vi "Translate Weight Calibration.vi"(10 "Known Weight Tool Coordinates":T1, 11 "Known HDI Fiducials Coordinates":T2) -> (1 "brass piece rotation":dbl, 2 "Orient3d String":string, 3 "Vec3d String":string)   [LabVIEW 2011]
uses:
  Shared Components/Vec3d Class/Vec3d Class.lvclass
  Shared Components/Orient3d Class/Orient3d Class.lvclass
panel:
  out "Pos Z":dbl
  out "Pos Y":dbl
  out "Pos X":dbl
  out "orient w":dbl
  out "orient z":dbl
  out "orient y":dbl
  out "orient x":dbl
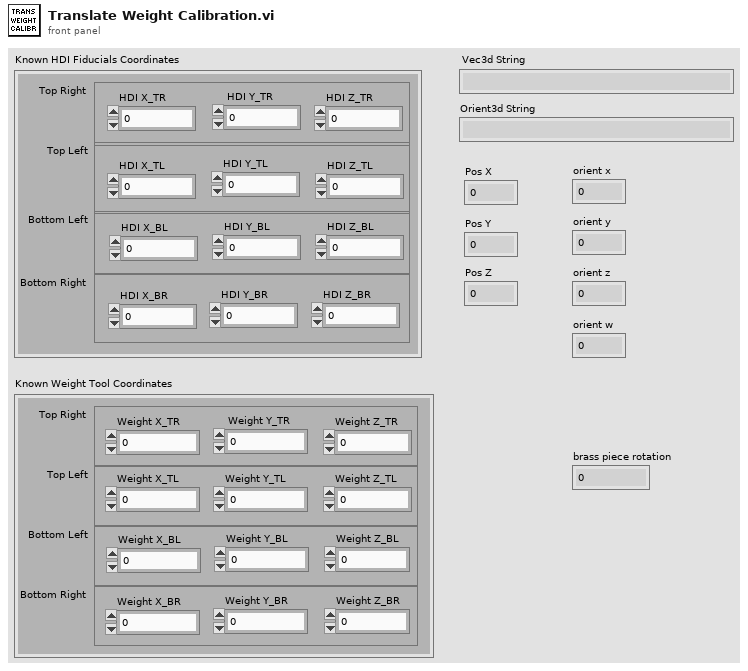
[diagram p1: front panel]
types:
  T1 = cluster{"Top Right":cluster{"Weight X_TR":dbl, " Weight Y_TR":dbl, "Weight Z_TR":dbl}, "Top Left":cluster{"Weight X_TL":dbl, "Weight Y_TL":dbl, "Weight Z_TL":dbl}, "Bottom Left":cluster{"Weight X_BL":dbl, "Weight Y_BL":dbl, "Weight Z_BL":dbl}, "Bottom Right":cluster{"Weight X_BR":dbl, "Weight Y_BR":dbl, "Weight Z_BR":dbl}}
  T2 = cluster{"Top Right":cluster{"HDI X_TR":dbl, " HDI Y_TR":dbl, "HDI Z_TR":dbl}, "Top Left":cluster{"HDI X_TL":dbl, "HDI Y_TL":dbl, "HDI Z_TL":dbl}, "Bottom Left":cluster{"HDI X_BL":dbl, "HDI Y_BL":dbl, "HDI Z_BL":dbl}, "Bottom Right":cluster{"HDI X_BR":dbl, "HDI Y_BR":dbl, "HDI Z_BR":dbl}}
  T3 = cluster{"Weight X_TR":dbl, " Weight Y_TR":dbl, "Weight Z_TR":dbl}
  T4 = cluster{"Weight X_TL":dbl, "Weight Y_TL":dbl, "Weight Z_TL":dbl}
  T5 = cluster{"Weight X_BL":dbl, "Weight Y_BL":dbl, "Weight Z_BL":dbl}
  T6 = cluster{"Weight X_BR":dbl, "Weight Y_BR":dbl, "Weight Z_BR":dbl}
  T7 = cluster{"HDI X_TR":dbl, " HDI Y_TR":dbl, "HDI Z_TR":dbl}
  T8 = cluster{"HDI X_TL":dbl, "HDI Y_TL":dbl, "HDI Z_TL":dbl}
  T9 = cluster{"HDI X_BL":dbl, "HDI Y_BL":dbl, "HDI Z_BL":dbl}
  T10 = cluster{"HDI X_BR":dbl, "HDI Y_BR":dbl, "HDI Z_BR":dbl}
  T11 = typedef "Position_Orientation.ctl" = cluster{"Center":refnum<class "Vec3d Class.lvclass">, "Orientation":refnum<class "Orient3d Class.lvclass">}
  T12 = typedef "Quaternion.ctl" = cluster{"x":dbl, "y":dbl, "z":dbl, "w":dbl}
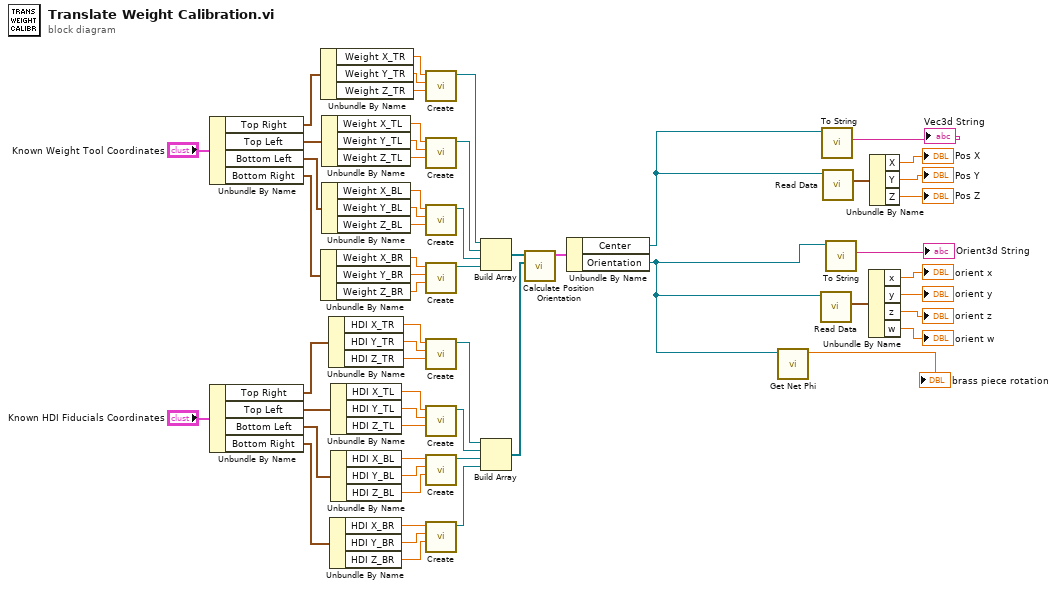
[diagram p0: block diagram]
diagram:
  n1 = Unbundle By Name("Known Weight Tool Coordinates") -> ("Top Right"=w22:T3, "Top Left"=w21:T4, "Bottom Left"=w20:T5, "Bottom Right"=w19:T6)
  n2 = Unbundle By Name("Known HDI Fiducials Coordinates") -> ("Top Right"=w39:T7, "Top Left"=w35:T8, "Bottom Left"=w28:T9, "Bottom Right"=w24:T10)
  n3 = Unbundle By Name(w22) -> ("Weight X_TR"=w18:dbl, "Weight Y_TR"=w17:dbl, "Weight Z_TR"=w16:dbl)
  n4 = Unbundle By Name(w19) -> ("Weight X_BR"=w9:dbl, "Weight Y_BR"=w8:dbl, "Weight Z_BR"=w7:dbl)
  n5 = Unbundle By Name(w21) -> ("Weight X_TL"=w15:dbl, "Weight Y_TL"=w14:dbl, "Weight Z_TL"=w13:dbl)
  n6 = Unbundle By Name(w20) -> ("Weight X_BL"=w12:dbl, "Weight Y_BL"=w11:dbl, "Weight Z_BL"=w10:dbl)
  n7 = Unbundle By Name(w39) -> ("HDI X_TR"=w38:dbl, "HDI Y_TR"=w37:dbl, "HDI Z_TR"=w36:dbl)
  n8 = Unbundle By Name(w24) -> ("HDI X_BR"=w27:dbl, "HDI Y_BR"=w26:dbl, "HDI Z_BR"=w25:dbl)
  n9 = Unbundle By Name(w35) -> ("HDI X_TL"=w34:dbl, "HDI Y_TL"=w33:dbl, "HDI Z_TL"=w32:dbl)
  n10 = Unbundle By Name(w28) -> ("HDI X_BL"=w31:dbl, "HDI Y_BL"=w30:dbl, "HDI Z_BL"=w29:dbl)
  n11 = call "Create.vi"("Z"=w16, "Y"=w17, "X"=w18) -> ("Vec3d Class out"=w55:refnum<class "Vec3d Class.lvclass">)  [unwired: 7 in, 1 out]
  n12 = call "Create.vi"("Z"=w13, "Y"=w14, "X"=w15) -> ("Vec3d Class out"=w54:refnum<class "Vec3d Class.lvclass">)  [unwired: 7 in, 1 out]
  n13 = call "Create.vi"("Z"=w10, "Y"=w11, "X"=w12) -> ("Vec3d Class out"=w53:refnum<class "Vec3d Class.lvclass">)  [unwired: 7 in, 1 out]
  n14 = call "Create.vi"("Z"=w7, "Y"=w8, "X"=w9) -> ("Vec3d Class out"=w51:refnum<class "Vec3d Class.lvclass">)  [unwired: 7 in, 1 out]
  n15 = call "Create.vi"("Z"=w36, "Y"=w37, "X"=w38) -> ("Vec3d Class out"=w59:refnum<class "Vec3d Class.lvclass">)  [unwired: 7 in, 1 out]
  n16 = call "Create.vi"("Z"=w32, "Y"=w33, "X"=w34) -> ("Vec3d Class out"=w58:refnum<class "Vec3d Class.lvclass">)  [unwired: 7 in, 1 out]
  n17 = call "Create.vi"("Z"=w29, "Y"=w30, "X"=w31) -> ("Vec3d Class out"=w57:refnum<class "Vec3d Class.lvclass">)  [unwired: 7 in, 1 out]
  n18 = call "Create.vi"("Z"=w25, "Y"=w26, "X"=w27) -> ("Vec3d Class out"=w52:refnum<class "Vec3d Class.lvclass">)  [unwired: 7 in, 1 out]
  n19 = Build Array(w55, w54, w53, w51) -> (w50:refnum<class "Vec3d Class.lvclass">[])
  n20 = Build Array(w59, w58, w57, w52) -> (w56:refnum<class "Vec3d Class.lvclass">[])
  n21 = call "Calculate Position Orientation.vi"("Measured Global Positions"=w56, "Known Local Positions"=w50) -> ("PositionOrientation"=w49:T11)  [unwired: 7 in, 2 out]
  n22 = Unbundle By Name(w49) -> ("Center"=w2:refnum<class "Vec3d Class.lvclass">, "Orientation"=w1:refnum<class "Orient3d Class.lvclass">)
  n23 = call "Get Net Phi.vi"("Orient3d"=w1) -> ("phi(deg)"=→"brass piece rotation":dbl)  [unwired: 8 in, 2 out]
  n24 = call "Read Data.vi"("Orient3d in"=w1) -> ("Quaternion"=w48:T12)  [unwired: 8 in, 2 out]
  n25 = call "To String.vi"("Vec3d in"=w2) -> ("Vec3d String"=→"Vec3d String":string)  [unwired: 8 in, 2 out]
  n26 = call-dynamic "Read Data.vi"("Vec3d Class in"=w2) -> ("Data"=w3:cluster{"X":dbl, "Y":dbl, "Z":dbl})  [unwired: 8 in, 2 out]
  n27 = call "To String.vi"("Orient3d in"=w1) -> ("Orient3d String"=→"Orient3d String":string)  [unwired: 8 in, 2 out]
  n28 = Unbundle By Name(w48) -> ("x"=→"orient x":dbl, "y"=→"orient y":dbl, "z"=→"orient z":dbl, "w"=→"orient w":dbl)
  n29 = Unbundle By Name(w3) -> ("X"=→"Pos X":dbl, "Y"=→"Pos Y":dbl, "Z"=→"Pos Z":dbl)
